vi "Read_Field.vi"() -> ()   [LabVIEW 2013]
uses:
  <instrlib>/Mercury iXX/Public/Controls/Comms Transport Layer.ctl
  <instrlib>/Mercury iXX/Public/Controls/Serial Settings.ctl
  <instrlib>/Mercury iXX/Public/Controls/ISOBus Address.ctl
  <instrlib>/Mercury iXX/Public/Libraries/Magnet/Controls/Identifier.ctl
  <instrlib>/Mercury iXX/Public/Controls/Unit String.ctl
  <instrlib>/Mercury iXX/Public/Libraries/System/Open/Open System.vi
  <instrlib>/Mercury iXX/Public/Libraries/System/Read/Catalogue (Read).vi
  <instrlib>/Mercury iXX/Public/Libraries/Magnet/Open/Open Magnet Device.vi
  <instrlib>/Mercury iXX/Public/Libraries/Magnet/Signals/Read/Field (Read).vi
  <instrlib>/Mercury iXX/Mercury iXX.lvlib
  <instrlib>/Mercury iXX/Public/Libraries/System.lvlib
  <instrlib>/Mercury iXX/Public/Libraries/Magnet.lvlib
panel:
  in  "stop":bool
  out "error out":errorcluster
  out "Unit":T1
  out "Field":dbl format="%.4g"
  in  "Device Identifier":T2="GRPZ"
  in  "ISOBUS address":T3=-1 caption="ISOBUS address (-1)"
  out "Devices":string[](array[string])
  in  "Clear Previous Connections (False)":bool
  in  "ID Query (True)":bool
  in  "Serial Configuration":T4={"Baud Rate"=9600, "Parity"=0, "Data Bits"=8, "Stop Bits"=10, "Flow Control"=0} {"Flow Control" items=["None", "XON/XOFF", "RTS/CTS", "XON/XOFF & RTS/CTS", "DTR/DSR", "XON/XOFF & DTR/DSR"]; "Stop Bits" items=["1.0"=10, "2.0"=20]; "Data Bits" items=["7"=7, "8"=8]; "Parity" items=["None", "Odd", "Even"]; "Baud Rate" items=["300"=300, "600"=600, "1200"=1200, "2400"=2400, "4800"=4800, "9600"=9600, "19200"=19200]}
  in  "Comms Layer":T5
  in  "IP Address":string
  in  "VISA resource name":refnum<visa-resource-name>
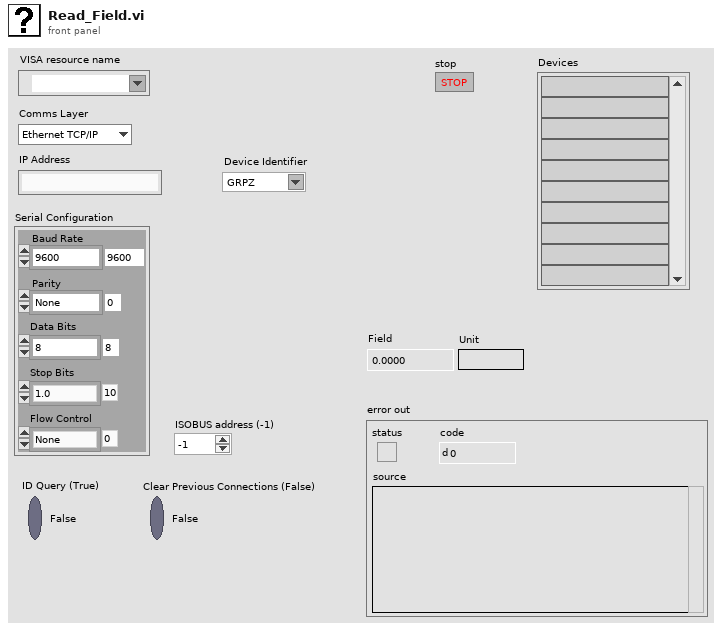
[diagram p1: front panel]
types:
  T1 = typedef "Mercury iXX.lvlib/Unit String.ctl" = string
  T2 = typedef "Mercury iXX.lvlib/Magnet.lvlib/Identifier.ctl" = string
  T3 = typedef "Mercury iXX.lvlib/ISOBus Address.ctl" = i32
  T4 = typedef "Mercury iXX.lvlib/Serial Settings.ctl" = cluster{"Baud Rate":u32, "Parity":u16, "Data Bits":u16, "Stop Bits":u16, "Flow Control":u16}
  T5 = typedef "Mercury iXX.lvlib/Comms Transport Layer.ctl" = enum16{"Ethernet TCP/IP", "USB", "ISOBus - RS-232", "GPIB"}
  T6 = typedef "Mercury iXX.lvlib/Mercury Reference.ctl" = cluster{"Comms":refnum<visa-resource-name>, "Device ID":string[], "Comms Layer":T5, "Command":string, "Query reference":T7}
  T7 = typedef "Mercury iXX.lvlib/Query Dynamic Reference.ctl" = refnum<vi>
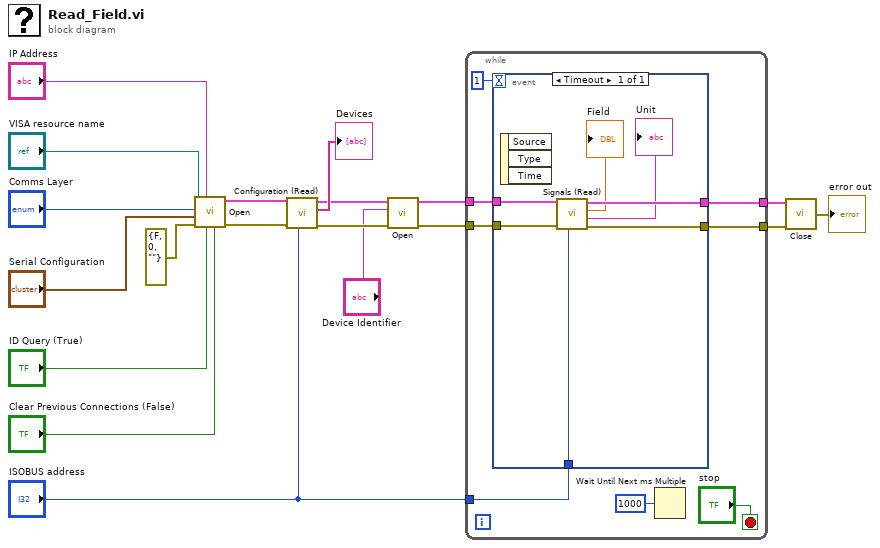
[diagram p0: block diagram]
diagram:
  n1 = call-poly <instrlib>:"Open.vi"("Clear Previous Connections (False)"="Clear Previous Connections (False)", "ID Query (True)"="ID Query (True)", "IP Address"="IP Address", "error in (no error)"=errorcluster {"status"=FALSE, "code"=0, "source"=""}, "Serial Configuration"="Serial Configuration", "Comms Layer"="Comms Layer", "VISA resource name"="VISA resource name") -> ("error out"=w11:errorcluster, "Mercury Reference Out"=w12:T6)  [unwired: 3 out]
  n2 = call-poly <instrlib>:"Configuration (Read).vi"("ISOBUS address"="ISOBUS address", "error in"=w11, "Mercury Reference In"=w12) -> ("error out"=w8:errorcluster, "Devices"=→"Devices":string[], "Mercury Reference Out"=w9:T6)  [unwired: 5 in, 1 out]
  n3 = call-poly <instrlib>:"Open.vi"("error in (no error)"=w8, "Device Identifier"="Device Identifier", "Mercury Reference In"=w9) -> ("error out"=w5:errorcluster, "Mercury Reference Out"=w6:T6)  [unwired: 7 in]
  n4 = while {
    tunnel: w6 -> [w27]
    tunnel: w5 -> [w26]
    tunnel: "ISOBUS address" -> [w25]
    tunnel: [w24] -> w3
    tunnel: [w23] -> w2
    stop <- "stop" stop-if-true
    n5 = event shown="[0] Timeout" {
      selector: _ -> [_]
      dyn-events: _ -> [_]
      timeout: 1 -> [_]
      tunnel: w27 -> [w34]
      tunnel: w26 -> [w33]
      tunnel: w25 -> [w32]
      tunnel: [w31] -> w24
      tunnel: [w30] -> w23
      event Timeout {
        n6 = event-data() -> ()  [unwired: 1 in, 3 out]
        n7 = call-poly <instrlib>:"Signals (Read).vi"("ISOBUS address"=w32, "error in"=w33, "Mercury Reference In"=w34) -> ("error out"=w30:errorcluster, "Unit"=→"Unit":T1, "Field"=→"Field":dbl, "Mercury Reference Out"=w31:T6)  [unwired: 4 in, 1 out]
      }
    }
    n8 = Wait Until Next ms Multiple(millisecond multiple=u32 1000) -> ()  [unwired: 1 out]
  }
  n9 = call <instrlib>:"Close.vi"("error in (no error)"=w2, "Mercury Reference"=w3) -> ("error out"=→"error out":errorcluster)  [unwired: 9 in]
